vi "Update UI Project.vi"(8 "error in (no error)":errorcluster, 10 "New Name":string, 11 "Template Project Path":path) -> (0 "error out":errorcluster)   [LabVIEW 2021, in "Plugin Generator.lvlib"]
uses:
  Plugin Generator.lvlib
  <vilib>/CIF Foundation/CIF LabVIEW Scripting/LV Scripting/LV Scripting Utilities.lvlib
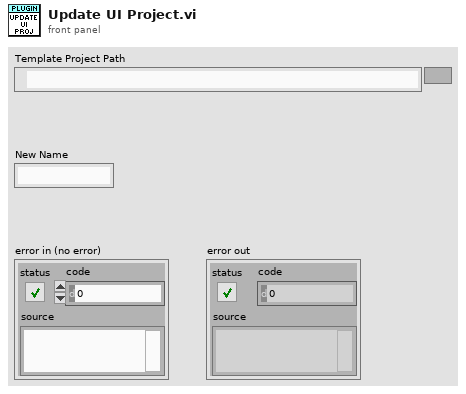
[diagram p1: front panel]
types:
  T1 = cluster{"Library Name":string, "Update Folder Name":bool}[]
  T2 = typedef "LV Scripting Utilities.lvlib/Target References.ctl" = cluster{"Target Reference":refnum<vi>, "VI References":refnum<vi>[], "Library References":refnum<vi>[], "Build References":refnum<vi>[]}
  T3 = typedef "LV Scripting Utilities.lvlib/Library Map.ctl" = map{string, refnum<vi>}
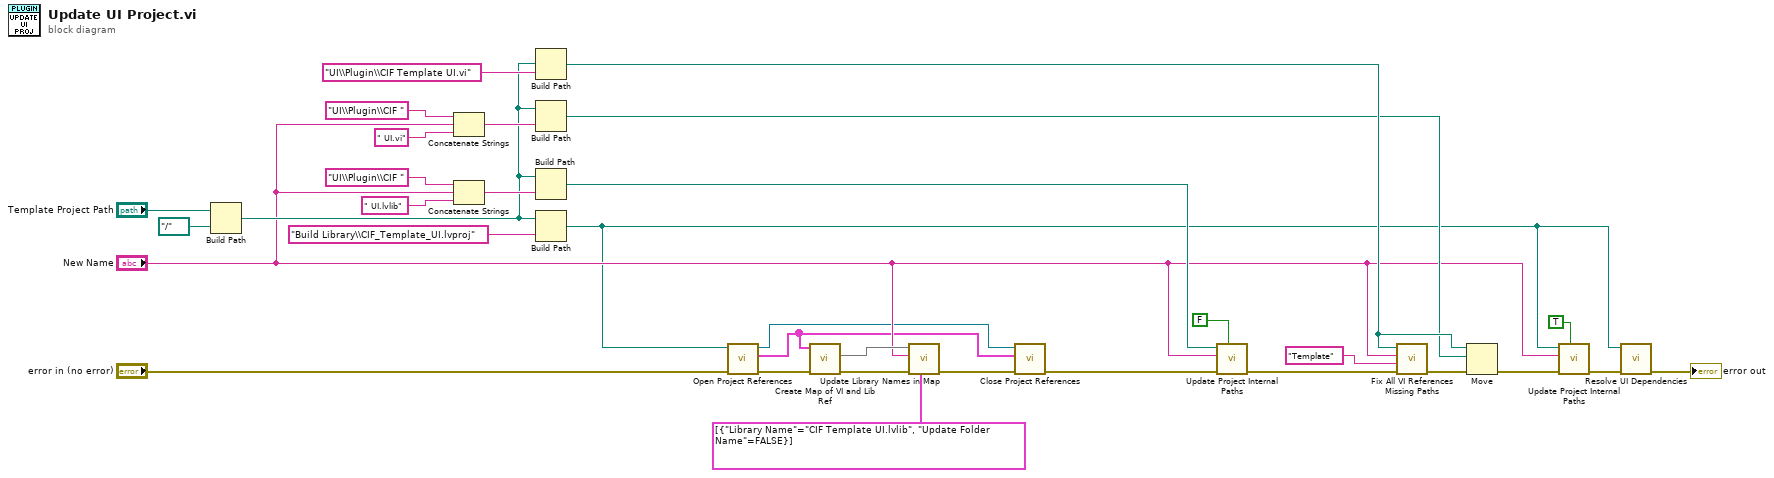
[diagram p0: block diagram]
diagram:
  n1 = Build Path(base path="Template Project Path", name or relative path=path "../..") -> (appended path=w13:path)
  n2 = Concatenate Strings("UI\\Plugin\\CIF " ("Class Name"), "New Name", " UI.vi" ("Class Name")) -> (w26:string)
  n3 = Concatenate Strings("UI\\Plugin\\CIF " ("Class Name"), "New Name", " UI.lvlib" ("Class Name")) -> (w14:string)
  n4 = Build Path(base path=w13, name or relative path="UI\\Plugin\\CIF Template UI.vi" ("Class Name")) -> (appended path=w29:path)
  n5 = Build Path(base path=w13, name or relative path=w26) -> (appended path=w25:path)
  n6 = Build Path(base path=w13, name or relative path=w14) -> (appended path=w21:path)
  n7 = Build Path(base path=w13, name or relative path="Build Library\\CIF_Template_UI.lvproj" ("Class Name")) -> (appended path=w1:path)
  n8 = call <vilib>:"Open Project References.vi"("error in"="error in (no error)", "Project Path"=w1) -> ("error out"=w6:errorcluster, "VI, Library, and Build References"=w3:T2[], "Project Reference"=w2:refnum<vi>)  [unwired: 7 in]
  n9 = call <vilib>:"Create Map of VI and Lib Ref.vi"("error in"=w6, "VI, Library, and Build References"=w3) -> ("error out"=w18:errorcluster, "Library Map"=w19:T3)  [unwired: 6 in, 2 out]
  n10 = call <vilib>:"Update Library Names in Map.vi"("Libraries"=T1 [{"Library Name"="CIF Template UI.lvlib", "Update Folder Name"=FALSE}], "error in"=w18, "New Subname"="New Name", "Library Map"=w19) -> ("error out"=w5:errorcluster)  [unwired: 6 in, 1 out]
  n11 = call <vilib>:"Close Project References.vi"("error in"=w5, "VI, Library, and Build References"=w3, "Project Reference"=w2) -> ("error out"=w4:errorcluster)  [unwired: 8 in]
  n12 = call <vilib>:"Update Project Internal Paths.vi"("Rename Project"=FALSE, "error in (no error)"=w4, "New Subname"="New Name", "Project Path"=w21) -> ("error out"=w23:errorcluster)  [unwired: 7 in]
  n13 = call <vilib>:"Fix All VI References Missing Paths.vi"("error in (no error)"=w23, "Replace Subname"="Template" ("Subname to Replace"), "New Subname"="New Name", "VI Path"=w29) -> ("error out"=w22:errorcluster)  [unwired: 7 in]
  n14 = Move(source path=w29, error in=w22, 10:w25) -> (error out=w24:errorcluster)  [unwired: 2 in, 2 out]
  n15 = call <vilib>:"Update Project Internal Paths.vi"("Rename Project"=TRUE, "error in (no error)"=w24, "New Subname"="New Name", "Project Path"=w1) -> ("error out"=w9:errorcluster)  [unwired: 7 in]
  n16 = call "Resolve UI Dependencies.vi"("error in"=w9, "Template Project Path"=w1) -> ("error out"=→"error out":errorcluster)  [unwired: 9 in]
